vi "stageGoLeft.vi"() -> ()   [LabVIEW 2016]
uses:
  <vilib>/Instr/_visa.llb/VISA Configure Serial Port (Instr).vi
panel:
  out "Moving":bool
  in  "Stage Position":string
  in  "Step length (um)":dbl=100.0
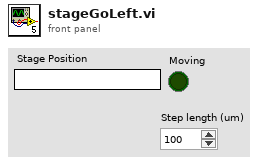
[diagram p1: front panel]
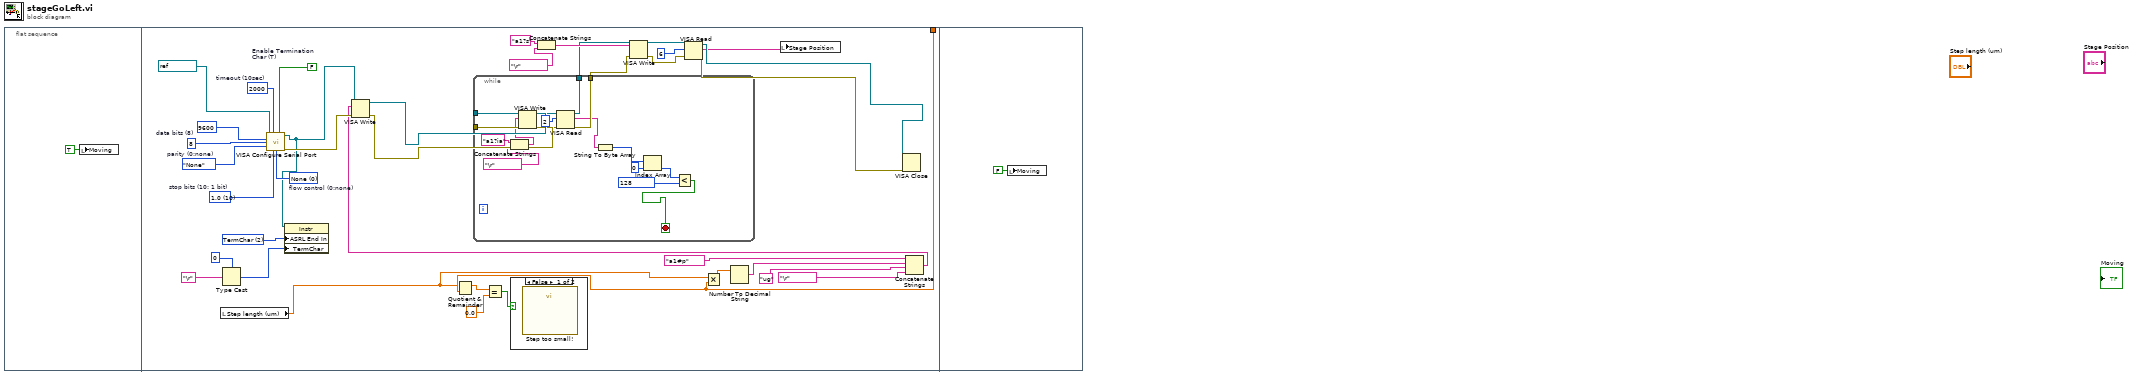
[diagram p0: block diagram]
diagram:
  n1 = flat-sequence {
    tunnel: _ -> [w3]
    frame #0 {
      n2 = local write "Moving"(TRUE ("Moving")) -> ()
    }
    frame #1 {
      w9 = u16 2 items=["None", "Last Bit", "TermChar"] ("Serial Settings:End Mode for Reads")
      w32 = u16 0 items=["None", "XON/XOFF", "RTS/CTS", "XON/XOFF & RTS/CTS", "DTR/DSR", "XON/XOFF & DTR/DSR"]  # flow control (0:none)
      w31 = u16 10 items=["1.0"=10, "1.5"=15, "2.0"=20]  # stop bits (10: 1 bit)
      w30 = FALSE  # Enable Termination Char (T)
      w29 = u32 2000  # timeout (10sec)
      w28 = enum16{"None", "Odd", "Even", "Mark", "Space"}."None"  # parity (0:none)
      w27 = u16 8  # data bits (8)
      n3 = local read "Step length (um)"() -> (w2:dbl)
      n4 = Type Cast(type=u8 0, x="\r") -> (*(type *) &x=w11:u8)
      n5 = call-poly "VISA Configure Serial Port"("VISA resource name"=refnum<visa-resource-name> "COM4", "timeout (10sec)"=w29, "Enable Termination\nChar (T)"=w30, "baud rate (9600)"=u32 9600, "data bits (8)"=w27, "parity (0:none)"=w28, "stop bits (10: 1 bit)"=w31, "flow control (0:none)"=w32) -> ("VISA resource name out"=w8:refnum<visa-resource-name>, "error out"=w39:errorcluster)  [unwired: 6 in]
      n6 = property class="Instr"(reference=w8, "ASRL End In"=w9, "TermChar"=w11) -> ()  [unwired: 1 in, 2 out]
      n7 = Quotient & Remainder(x=w2, y=w3) -> (x-y*floor(x/y)=w6:dbl)  [unwired: 1 out]
      n8 = Equal?(x=w6, y=0.0) -> (x = y?=w4:bool)
      n9 = case shown="False" w4 {
        frame False {
          n10 = call "Step too small!"() -> ()  [unwired: 18 in, 2 out]
        }
        frame True {
        }
      }
      n11 = Concatenate Strings("a1?s" ("write buffer"), "\r" ("write buffer")) -> (w23:string)
      n12 = Multiply(x=w2, y=w3) -> (x*y=w7:dbl)
      n13 = Number To Decimal String(number=w7) -> (decimal integer string=w35:string)  [unwired: 1 in]
      n14 = Concatenate Strings("a1#p" ("string"), w35, "ug" ("string"), "\r" ("write buffer")) -> (w34:string)
      n15 = VISA Write(VISA resource name=w8, write buffer=w34, error in (no error)=w39) -> (VISA resource name out=w15:refnum<visa-resource-name>, error out=w14:errorcluster)  [unwired: 1 out]
      n16 = while {
        tunnel: w15 -> [w55]
        tunnel: w14 -> [w54]
        tunnel: [w47] -> w20
        tunnel: [w46] -> w19
        stop <- w40 stop-if-true
        n17 = Concatenate Strings("a1?ia" ("write buffer"), "\r" ("write buffer")) -> (w51:string)
        n18 = VISA Write(VISA resource name=w55, write buffer=w51, error in (no error)=w54) -> (VISA resource name out=w50:refnum<visa-resource-name>, error out=w49:errorcluster)  [unwired: 1 out]
        n19 = VISA Read(VISA resource name=w50, byte count=u32 2, error in (no error)=w49) -> (VISA resource name out=w47:refnum<visa-resource-name>, read buffer=w45:string, error out=w46:errorcluster)  [unwired: 1 out]
        n20 = String To Byte Array(string=w45) -> (unsigned byte array=w44:u8[])
        n21 = Index Array(array=w44, index=0) -> (element=w42:u8)
        n22 = Less?(x=w42, y=u8 128) -> (x < y?=w40:bool)
      }
      n23 = VISA Write(VISA resource name=w20, write buffer=w23, error in (no error)=w19) -> (VISA resource name out=w24:refnum<visa-resource-name>, error out=w13:errorcluster)  [unwired: 1 out]
      n24 = VISA Read(VISA resource name=w24, byte count=u32 6, error in (no error)=w13) -> (VISA resource name out=w17:refnum<visa-resource-name>, read buffer=w16:string, error out=w18:errorcluster)  [unwired: 1 out]
      n25 = local write "Stage Position"(w16) -> ()
      n26 = VISA Close(VISA resource name=w17, error in (no error)=w18) -> ()  [unwired: 1 out]
    }
    frame #2 {
      n27 = local write "Moving"(FALSE ("Moving")) -> ()
    }
  }
